vi "getPackageLicense.vi"(8 "error":errorcluster, 10 "pckg":string, 11 "connection ID":refnum<k5>) -> (0 "error out":errorcluster, 2 "string":string, 3 "connection ID out":refnum<k5>)   [LabVIEW 2016, in "sen_api.lvlib"]
doc: "Get the license for a specific package."
uses:
  sen_api.lvlib
panel:
  out "jsonRespIn":string
  out "JSON-response":string="{\"jsonrpc\":\"2.0\",\"method\":\"\",\"params\":[5,1.245,true,\"name\"],\"id\":\"1\"}"
  out "JSON request":string
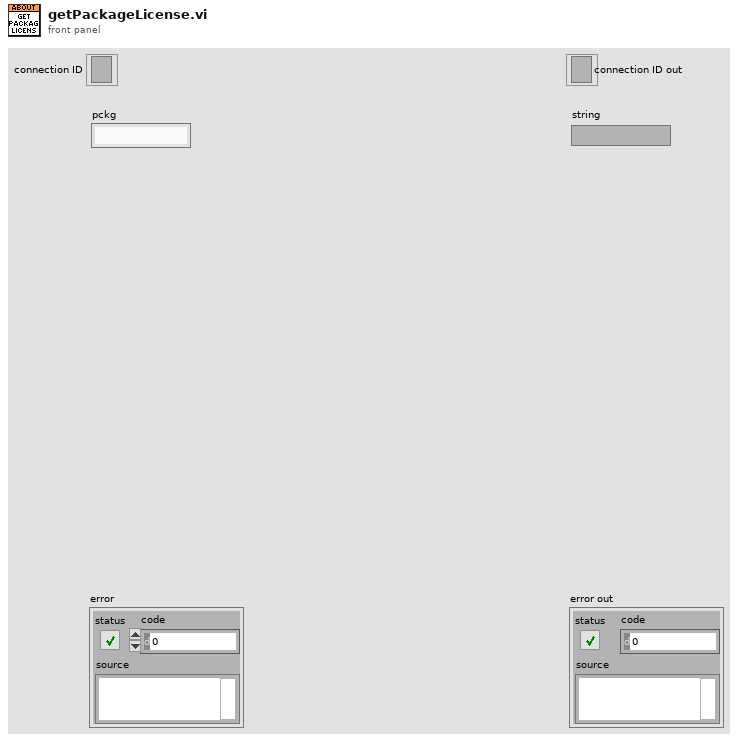
[diagram p1: front panel]
types:
  T1 = cluster{"jsonrpc":string, "method":string, "params":string[], "id":string, "api":i32, "pid":string}
  T2 = enum16{"Standard", "Buffered", "CRLF", "Immediate"}
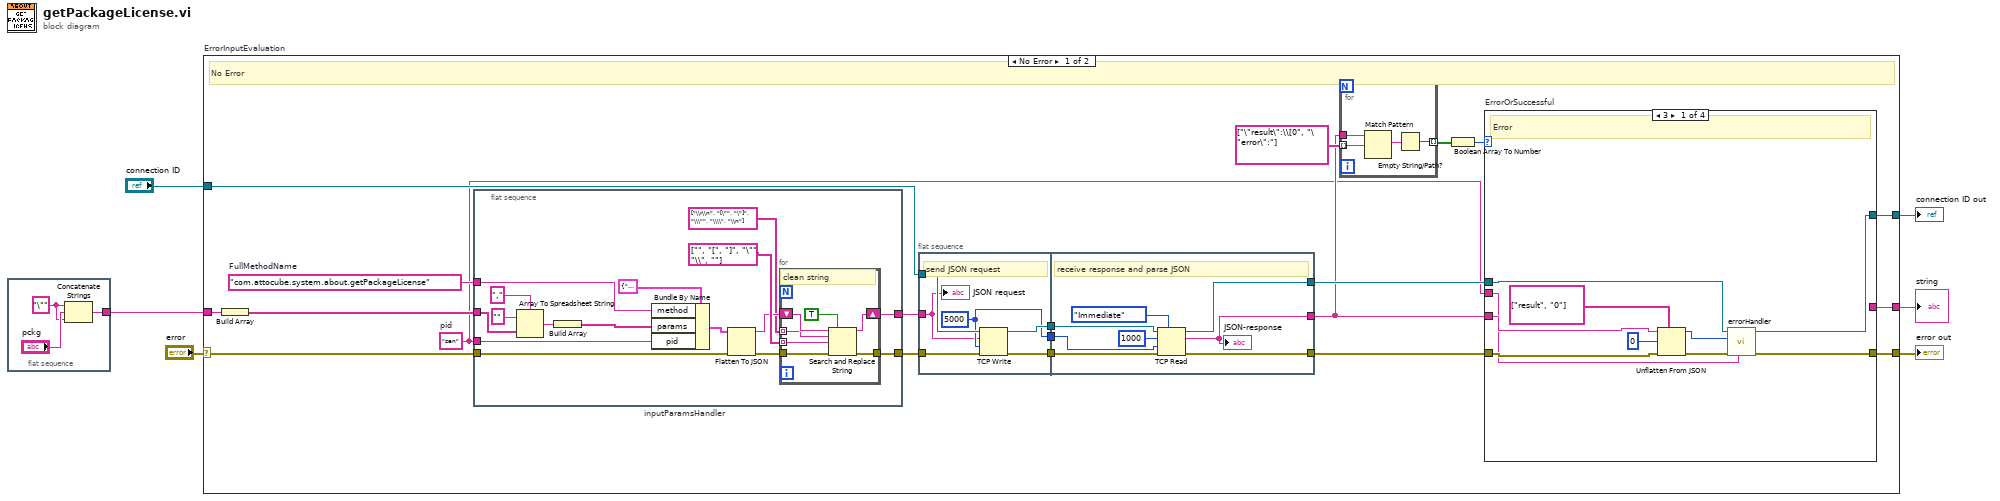
[diagram p0: block diagram]
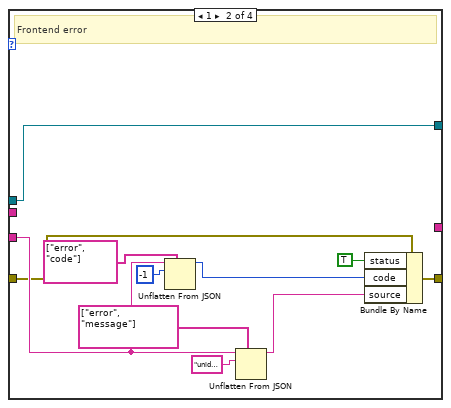
[diagram p2: hidden frame]
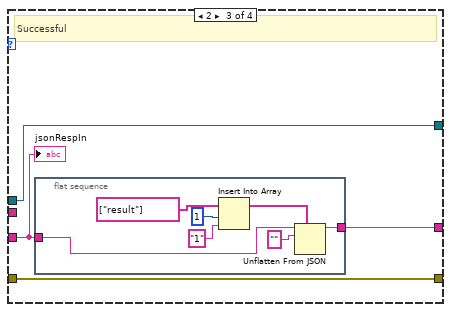
[diagram p3: hidden frame]
diagram:
  n1 = flat-sequence "in_string" {
    tunnel: [w8] -> w2
    frame #0 {
      w7 = "\"" ("string")
      n2 = Concatenate Strings(w7, "pckg", w7) -> (w8:string)
    }
  }
  n3 = case "ErrorInputEvaluation" shown="No Error" "error" {
    selector: "error" -> [w16 w105]
    tunnel: "connection ID" -> [w26 w106]
    tunnel: [w18 w105] -> w5
    tunnel: [w19 w106] -> w4
    tunnel: w2 -> [w11 _]
    tunnel: [w10 _] -> w1
    frame No Error {
      w12 = "sen"  # pid
      w17 = "com.attocube.system.about.getPackageLicense"  # FullMethodName
      # "No Error"
      n4 = Build Array ("ParametersArrayString")(w11) -> (w15:string[])
      n5 = flat-sequence "inputParamsHandler" {
        tunnel: [w33] -> w14
        tunnel: w15 -> [w40]
        tunnel: w16 -> [w38]
        tunnel: [w35] -> w13
        tunnel: w17 -> [w41]
        tunnel: w12 -> [w30]
        frame #0 {
          n6 = Array To Spreadsheet String(delimiter (Tab)=",", array=w40, 3:"" ("format string")) -> (spreadsheet string=w43:string)
          n7 = Build Array "Build Array"(w43) -> (w39:string[])
          n8 = Bundle By Name(cluster=T1 {"jsonrpc"="2.0", "method"="com.attocube.amc.res.setRESReadOutFreq", "params"=[], "id"="1", "api"=2, "pid"=""}, "method"=w41, "params"=w39, "pid"=w30) -> (w42:T1)
          n9 = Flatten To JSON(anything=w42, error in (no error)=w38) -> (JSON string=w34:string, 11:w36:errorcluster)  [unwired: 1 in]
          n10 = for {
            tunnel: string[] ["\\r\\n", "[\"", "\"]", "\\\"", "\\\\", "\\n"] ("search string") -> [w49] mode=indexing
            tunnel: string[] ["", "[", "]", "\"", "\\", ""] ("replace string (\"\")") -> [w48] mode=indexing
            shift-right: [w51] -> w33
            shift-left: w34 -> [w50]
            tunnel: w36 -> [w47]
            tunnel: [w46] -> w35
            # "clean string"
            n11 = Search and Replace String(replace all?=TRUE ("replace all? (F)"), input string=w50, search string=w49, replace string=w48, error in=w47) -> (result string=w51:string, error out=w46:errorcluster)  [unwired: 3 in, 2 out]
          }
        }
      }
      n12 = flat-sequence {
        tunnel: w26 -> [w96]
        tunnel: [w94] -> w29
        tunnel: [w95] -> w28
        tunnel: w13 -> [w91]
        tunnel: [w93] -> w27
        tunnel: w14 -> [w92]
        tunnel: [w100] -> w22
        tunnel: w29 -> [w102]
        tunnel: w28 -> [w101]
        tunnel: [w98] -> w21
        tunnel: w27 -> [w99]
        tunnel: [w97] -> w20
        frame #0 {
          w93 = 5000 ("timeout ms (25000)")
          # "send JSON request"
          n13 = TCP Write(connection ID=w96, data in=w92, error in (no error)=w91, 9:w93) -> (connection ID out=w94:refnum<k5>, error out=w95:errorcluster)  [unwired: 1 out]
          "JSON request" <- w92
        }
        frame #1 {
          # "receive response and parse JSON"
          n14 = TCP Read(connection ID=w102, bytes to read=1000, error in (no error)=w101, 7:T2."Immediate" ("mode (standard)"), 9:w99) -> (connection ID out=w100:refnum<k5>, data out=w97:string, error out=w98:errorcluster)
          "JSON-response" <- w97
        }
      }
      n15 = for {
        tunnel: string[] ["\"result\":\\[0", "\"error\":"] ("path") -> [w55] mode=indexing
        tunnel: [w53] -> w24 mode=indexing
        tunnel: w20 -> [w56]
        n16 = Match Pattern(string=w56, regular expression=w55) -> (match substring=w54:string)  [unwired: 1 in, 3 out]
        n17 = Empty String/Path?(string/path=w54) -> (empty?=w53:bool)
      }
      n18 = Boolean Array To Number(Boolean array=w24) -> (number=w23:u32)
      n19 = case "ErrorOrSuccessful" shown="3" w23 {
        tunnel: w20 -> [w60 w69 w79 _]
        tunnel: w22 -> [w64 w67 w81 w90]
        tunnel: [w62 w67 w81 w90] -> w19
        tunnel: [w63 w70 w80 w89] -> w18
        tunnel: w21 -> [w66 w68 w80 w89]
        tunnel: w12 -> [w57 _ _ _]
        tunnel: [_ _ w78 _] -> w10
        frame 3 {
          # "Error"
          n20 = Unflatten From JSON(path=string[] ["result", "0"], JSON string=w60, type and defaults=0, error in (no error)=w66) -> (value=w58:i32, error out=w65:errorcluster)  [unwired: 3 in]
          n21 = call "errorHandler.vi"("pid"=w57, "error in"=w65, "errNbr"=w58, "connection ID"=w64) -> ("error out 2"=w63:errorcluster, "connection ID out"=w62:refnum<k5>)  [unwired: 6 in]
        }
        frame 1 {
          # "Frontend error"
          n22 = Unflatten From JSON(path=string[] ["error", "code"], JSON string=w69, type and defaults=-1) -> (value=w76:i32)  [unwired: 4 in, 1 out]
          n23 = Unflatten From JSON(path=string[] ["error", "message"], JSON string=w69, type and defaults="unidentified error") -> (value=w77:string)  [unwired: 4 in, 1 out]
          n24 = Bundle By Name(cluster=w68, "status"=TRUE, "code"=w76, "source"=w77) -> (w70:errorcluster)
        }
        frame 2 {
          # "Successful"
          n25 = flat-sequence "out_string" {
            tunnel: w79 -> [w88]
            tunnel: [w82] -> w78
            frame #0 {
              n26 = Insert Into Array(array=string[] ["result"] ("path"), index=1, new element="1" ("idx")) -> (w85:string[])
              n27 = Unflatten From JSON(path=w85, JSON string=w88, type and defaults="") -> (value=w82:string)  [unwired: 4 in, 1 out]
            }
          }
          "jsonRespIn" <- w79
        }
        frame Default {
          # "NoResponse"
        }
      }
    }
    frame Error {
      # "Error"
    }
  }
  "error out" <- w5
  "connection ID out" <- w4
  "string" <- w1
